vi "util.ntr.dose-aux.vi"(11 "Unit Index":i32) -> (0 "Unit Water Temperature (UN_WT)":string, 1 "DO Dose pumps":string[](array[string]), 2 "Unit Water Level (UN_WL%d)":string, 3 "DO Unit Pumps":string[](array[string]), 4 "AIN SENSORS":string[](array[string]))   [LabVIEW 2024]
uses:
  controls/enum-ntr-io-format.ctl
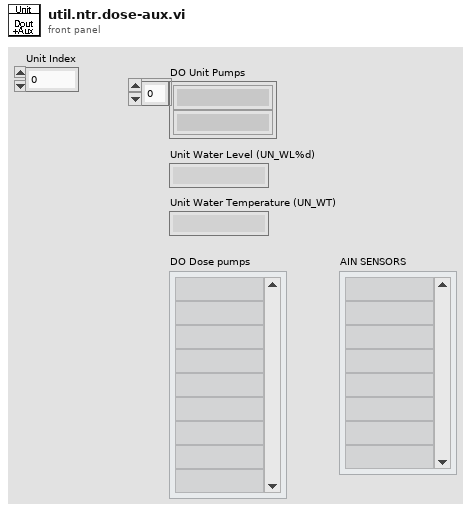
[diagram p1: front panel]
types:
  T1 = typedef "enum-ntr-io-format.ctl" = enum16{"UN_VLV%d", "UN_PMP%d", "UN_WL%d", "UN_PH", "UN_EC", "UN_ORP", "UN_WT", "UN_PH2", "UN_ALFA1", "UN_BETA1", "UN_ALFA2", "UN_BETA2", "UN_ACID", "UN_BASE", "UN_WATER", "UN_ORPMIX"}
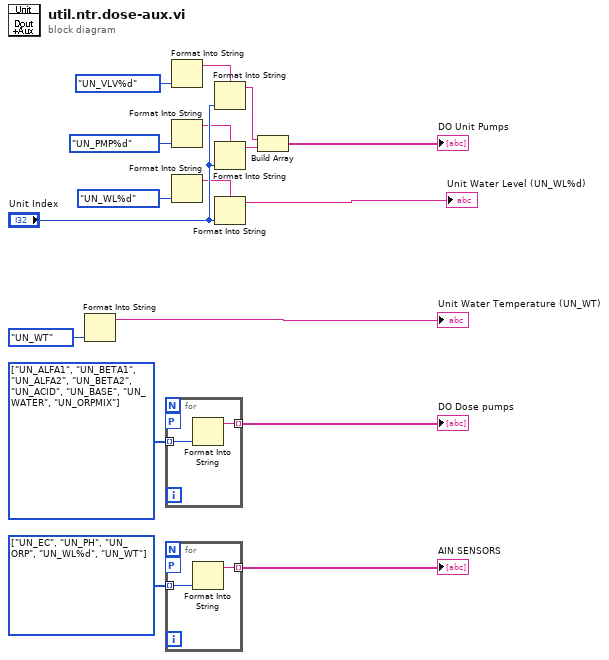
[diagram p0: block diagram]
diagram:
  w2 = T1[] [enum."UN_EC", enum."UN_PH", enum."UN_ORP", enum."UN_WL%d", enum."UN_WT"] items=["UN_VLV%d", "UN_PMP%d", "UN_WL%d", "UN_PH", "UN_EC", "UN_ORP", "UN_WT", "UN_PH2", "UN_ALFA1", "UN_BETA1", "UN_ALFA2", "UN_BETA2", "UN_ACID", "UN_BASE", "UN_WATER", "UN_ORPMIX"]
  w4 = T1[] [enum."UN_ALFA1", enum."UN_BETA1", enum."UN_ALFA2", enum."UN_BETA2", enum."UN_ACID", enum."UN_BASE", enum."UN_WATER", enum."UN_ORPMIX"] items=["UN_VLV%d", "UN_PMP%d", "UN_WL%d", "UN_PH", "UN_EC", "UN_ORP", "UN_WT", "UN_PH2", "UN_ALFA1", "UN_BETA1", "UN_ALFA2", "UN_BETA2", "UN_ACID", "UN_BASE", "UN_WATER", "UN_ORPMIX"]
  n1 = Format Into String(enum-ntr-io-format."UN_WT") -> (resulting string=→"Unit Water Temperature (UN_WT)":string)  [unwired: 3 in, 1 out]
  n2 = for {
    tunnel: w4 -> [w19] mode=indexing
    tunnel: [w18] -> w3 mode=indexing
    workers-P: _ -> [_]
    n3 = Format Into String(w19) -> (resulting string=w18:string)  [unwired: 3 in, 1 out]
  }
  "DO Dose pumps" <- w3
  n4 = for {
    tunnel: w2 -> [w21] mode=indexing
    tunnel: [w20] -> w1 mode=indexing
    workers-P: _ -> [_]
    n5 = Format Into String(w21) -> (resulting string=w20:string)  [unwired: 3 in, 1 out]
  }
  "AIN SENSORS" <- w1
  n6 = Format Into String(enum-ntr-io-format."UN_VLV%d") -> (resulting string=w11:string)  [unwired: 3 in, 1 out]
  n7 = Format Into String(enum-ntr-io-format."UN_PMP%d") -> (resulting string=w8:string)  [unwired: 3 in, 1 out]
  n8 = Format Into String(enum-ntr-io-format."UN_WL%d") -> (resulting string=w7:string)  [unwired: 3 in, 1 out]
  n9 = Format Into String(format string=w11, "Unit Index") -> (resulting string=w15:string)  [unwired: 2 in, 1 out]
  n10 = Format Into String(format string=w8, "Unit Index") -> (resulting string=w16:string)  [unwired: 2 in, 1 out]
  n11 = Format Into String(format string=w7, "Unit Index") -> (resulting string=→"Unit Water Level (UN_WL%d)":string)  [unwired: 2 in, 1 out]
  n12 = Build Array(w15, w16) -> (→"DO Unit Pumps":string[])
